vi "String.Append to Log, Limit Length.vi"(8 "Max Length":i32=1024 min=1 max=1000000 step=100, 9 "New Lines":string[](array[string]), 10 "New Line":string, 11 "Log In":string) -> (0 "Length":i32, 3 "Log Out":string)   [LabVIEW 2018]
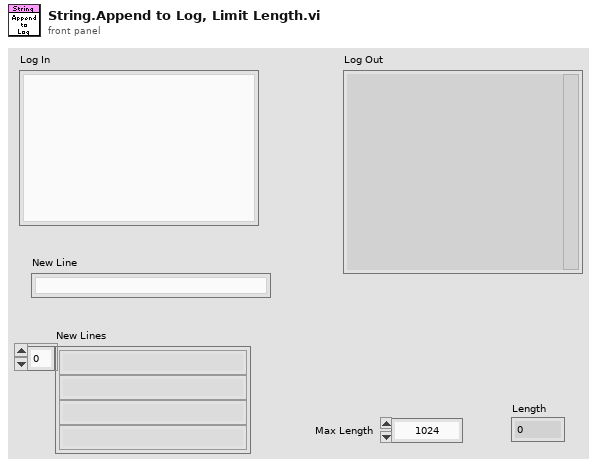
[diagram p1: front panel]
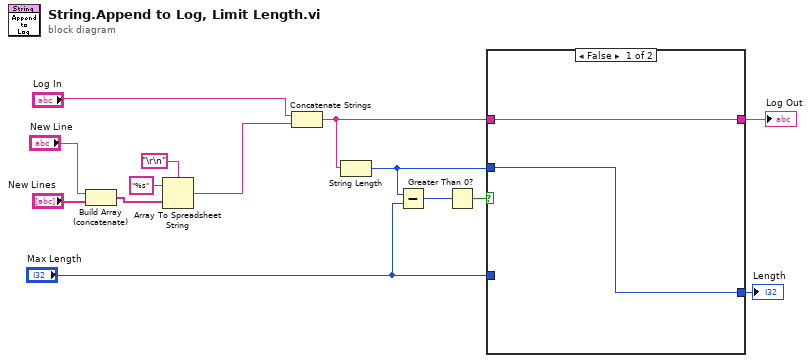
[diagram p0: block diagram]
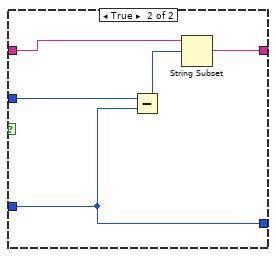
[diagram p2: hidden frame]
diagram:
  n1 = Build Array (concatenate)("New Line", "New Lines") -> (w8:string[])
  n2 = Array To Spreadsheet String(delimiter (Tab)="\r\n", array=w8, 3:"%s" ("format string")) -> (spreadsheet string=w12:string)
  n3 = Concatenate Strings("Log In", w12) -> (w6:string)
  n4 = String Length(string=w6) -> (length=w3:i32)
  n5 = Subtract(x=w3, y="Max Length") -> (x-y=w7:i32)
  n6 = Greater Than 0?(x=w7) -> (x > 0?=w4:bool)
  n7 = case shown="False" w4 {
    tunnel: w6 -> [w16 w21]
    tunnel: [w16 w18] -> w5
    tunnel: w3 -> [w15 w20]
    tunnel: [w15 w17] -> w2
    tunnel: "Max Length" -> [_ w17]
    frame False {
    }
    frame True {
      n8 = Subtract(x=w20, y=w17) -> (x-y=w19:i32)
      n9 = String Subset(string=w21, offset (0)=w19) -> (substring=w18:string)  [unwired: 1 in]
    }
  }
  "Log Out" <- w5
  "Length" <- w2
